vi "Debugging to XML.vi"() -> (0 "XML Data":string)   [LabVIEW 2013]
uses:
  Types/Debugging.ctl
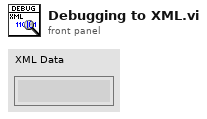
[diagram p1: front panel]
types:
  T1 = typedef "Debugging.ctl" = cluster{"In Place Debug Enabled":bool, "Version":string}
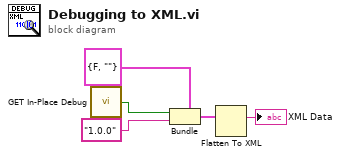
[diagram p0: block diagram]
diagram:
  n1 = call "GET In-Place Debug.vi"() -> ("In Place Debug Enabled"=w3:bool)
  n2 = Bundle(cluster=T1 {"In Place Debug Enabled"=FALSE, "Version"=""} ("Debugging"), "In Place Debug Enabled"=w3, "Version"="1.0.0") -> (w5:T1)
  n3 = Flatten To XML(anything=w5) -> (xml string=→"XML Data":string)
